vi "uncertainty.vi"(11 "Array":dbl[](array[numeric])) -> (0 "max inc":dbl, 3 "inc":dbl[](array[numeric]))   [LabVIEW 2021]
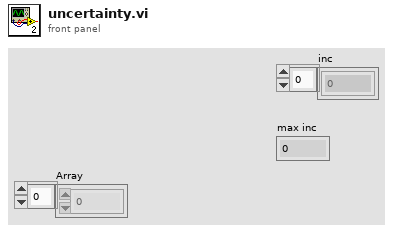
[diagram p1: front panel]
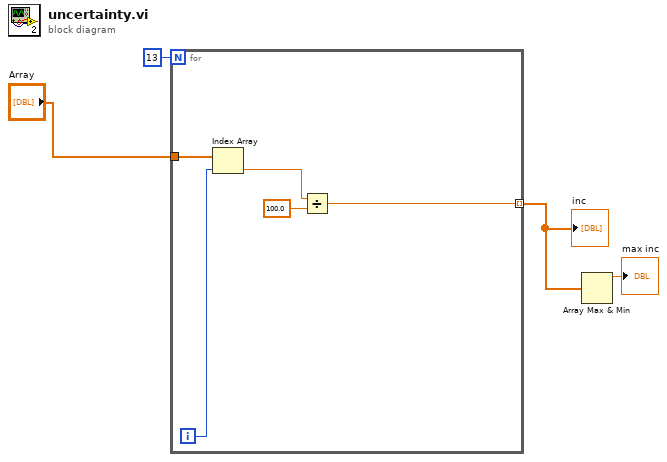
[diagram p0: block diagram]
diagram:
  n1 = for {
    N: 13 -> [_]
    tunnel: "Array" -> [w8]
    tunnel: [w6] -> w2 mode=indexing
    i -> [w5]
    n2 = Index Array(array=w8, index=w5) -> (element=w7:dbl)
    n3 = Divide(x=w7, y=100.0) -> (x/y=w6:dbl)
  }
  "inc" <- w2
  n4 = Array Max & Min(array=w2) -> (max value=→"max inc":dbl)  [unwired: 3 out]
